vi "Servo Connect if not.vi"(8 "error in":errorcluster, 10 "IP addresses":string[](array[string])) -> (0 "error out":errorcluster, 3 "Servo statuses":T1[](array[typedef]))   [LabVIEW 2021, in "Servo drive module.lvlib"]
doc: "Connect to all servo controllers with given IP addresses. Load their configuration and status.\nparams:\nIP addresess - an array of strings\nReturns:\nServo Statusses - an array of status cluser for each servo drive. Contains limiting constants and status variables."
uses:
  Servo drive module.lvlib
  ctl/Servo state.ctl
  ctl/Servo variables.ctl
  ctl/Servo constants.ctl
  ctl/Axis names.ctl
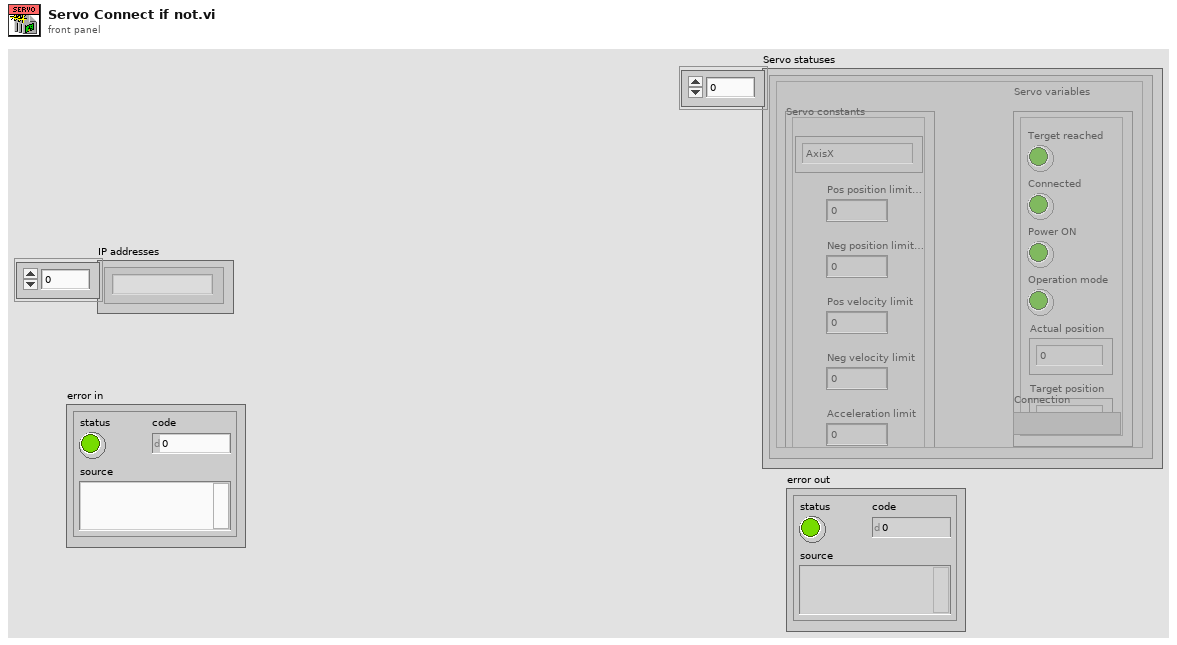
[diagram p1: front panel]
types:
  T1 = typedef "Servo drive module.lvlib/Servo state.ctl" = cluster{"Servo variables":T2, "Servo constants":T3, "Connection":variant}
  T2 = typedef "Servo drive module.lvlib/Servo variables.ctl" = cluster{"Terget reached":bool, "Connected":bool, "Power ON":bool, "Operation mode":bool, "Actual position":dbl, "Target position":dbl}
  T3 = typedef "Servo drive module.lvlib/Servo constants.ctl" = cluster{"Name":T4, "Pos position limit [mm]":dbl, "Neg position limit [mm]":dbl, "Pos velocity limit":dbl, "Neg velocity limit":dbl, "Acceleration limit":dbl}
  T4 = typedef "Servo drive module.lvlib/Axis names.ctl" = enum16{"Unknown", "AxisX", "AxisY", "AxisZ_left", "AxisZ_middle", "AxisZ_right"}
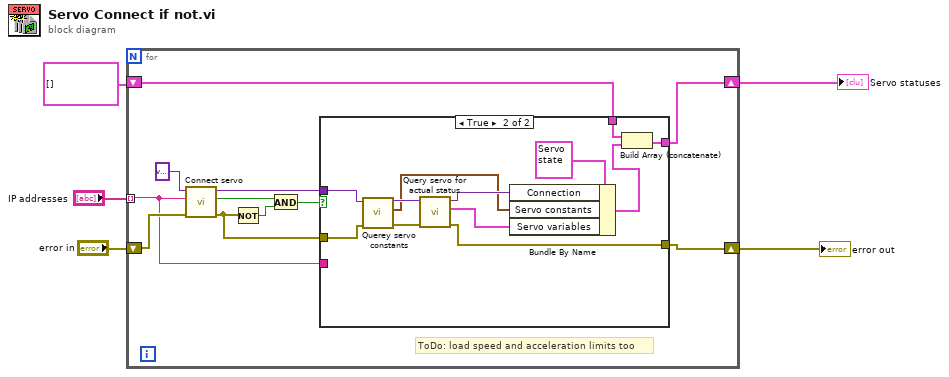
[diagram p0: block diagram]
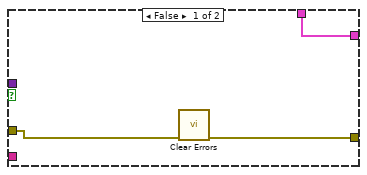
[diagram p2: hidden frame]
diagram:
  n1 = for {
    tunnel: "IP addresses" -> [w9] mode=indexing
    shift-right: [w15] -> w5
    shift-left: "error in" -> [w16]
    shift-right: [w8] -> w2
    shift-left: T1[] [] ("Array") -> [w6]
    # "ToDo: load speed and acceleration limits too"
    n2 = call "Connect servo.vi"("error in (no error)"=w16, "IP address"=w9, "Connection in"=variant ("Variant")) -> ("error out"=w10:errorcluster, "Is connected"=w11:bool, "Connection out"=w14:variant)  [unwired: 6 in]
    n3 = Not(x=w10) -> (.not. x?=w13:bool)
    n4 = And(x=w11, y=w13) -> (x .and. y?=w12:bool)
    n5 = case shown="True" w12 {
      tunnel: [w18 w25] -> w15
      tunnel: w14 -> [_ w30]
      tunnel: w10 -> [w19 w23]
      tunnel: w9 -> [_ _]
      tunnel: [w17 w20] -> w8
      tunnel: w6 -> [w17 w22]
      frame False {
        n6 = call <vilib>:"Clear Errors.vi"("error in (no error)"=w19) -> ("error out"=w18:errorcluster)  [unwired: 5 in, 1 out]
      }
      frame True {
        n7 = call "Querey servo constants.vi"("error in (no error)"=w23, "connection in"=w30) -> ("error out"=w24:errorcluster, "Servo constants"=w26:T3, "connection out"=w29:variant)  [unwired: 7 in]
        n8 = call "Query servo for actual status.vi"("error in (no error)"=w24, "connection in"=w29) -> ("error out"=w25:errorcluster, "Servo variables"=w27:T2, "connection out"=w28:variant)  [unwired: 7 in]
        n9 = Bundle By Name(cluster=T1 {"Servo variables"={"Terget reached"=FALSE, "Connected"=FALSE, "Power ON"=FALSE, "Operation mode"=FALSE, "Actual position"=0.0, "Target position"=0.0}, "Servo constants"={"Name"=enum."AxisX", "Pos position limit [mm]"=0.0, "Neg position limit [mm]"=0.0, "Pos velocity limit"=0.0, "Neg velocity limit"=0.0, "Acceleration limit"=0.0}, "Connection"=variant} ("Servo state"), "Connection"=w28, "Servo constants"=w26, "Servo variables"=w27) -> (w21:T1)
        n10 = Build Array (concatenate)(w22, w21) -> (w20:T1[])
      }
    }
  }
  "error out" <- w5
  "Servo statuses" <- w2
